vi "만도 소켓.vi"() -> ()   [LabVIEW 2023]
panel:
  out "array w/ subset deleted":dbl[](array[numeric])
  in  "Boolean":bool
  out "오차 각도":dbl
  out "x 교차점":dbl
  in  "stop":bool
  out "data out":string="99,99,0,0,0,0"
  out "전체 Array":dbl[](array[numeric])=[99.0, 99.0, 0.0, 0.0, 0.0, 0.0]
  out "빨간불":bool
  out "좌회전":bool
  out "직진":bool
  out "신호등 Array":dbl[](array[numeric])=[99.0, 99.0]
  out "생산자 FPS":dbl=111.11111111111111 format="%#_2g"
  out "error out":errorcluster
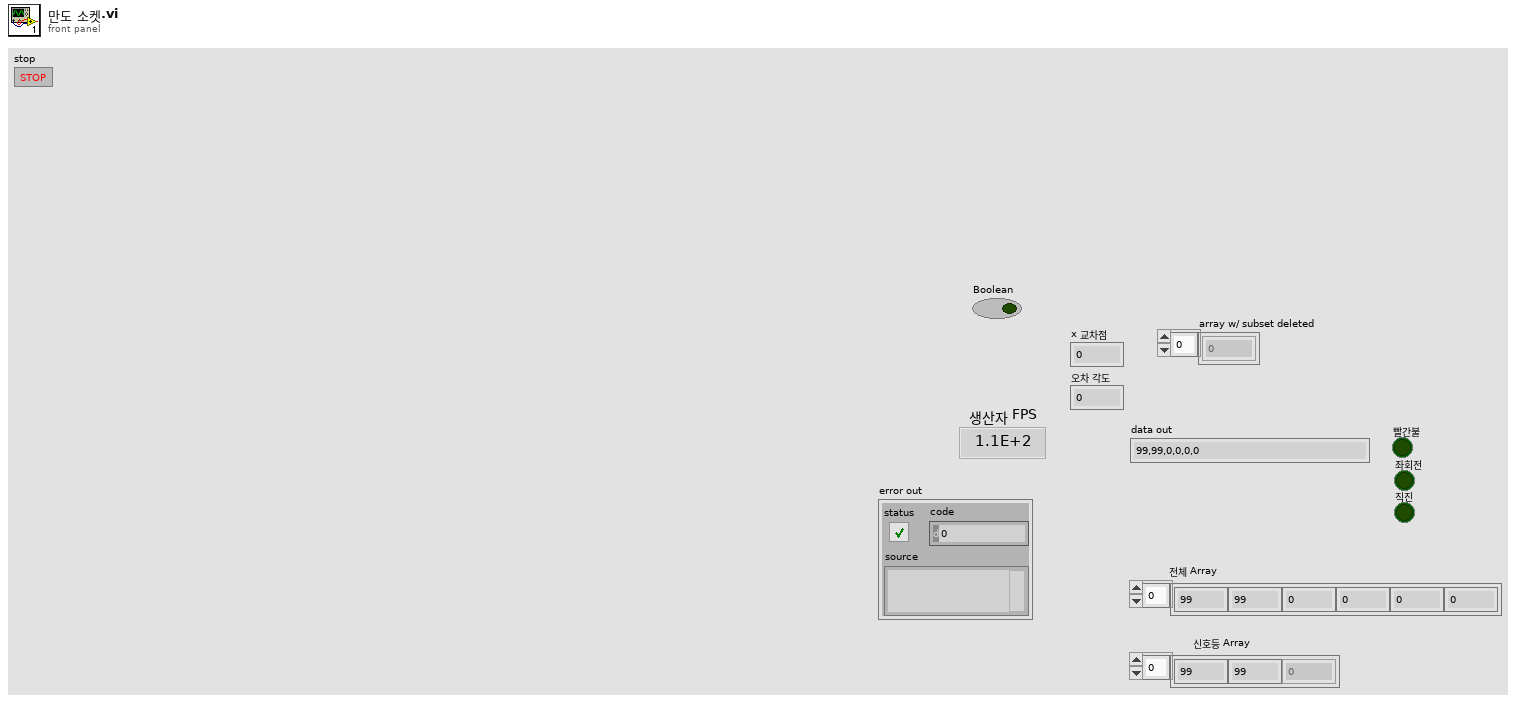
[diagram p1: front panel]
types:
  T1 = cluster{"빨간불":bool, "좌회전":bool, "직진":bool, "x 교차점":dbl, "오차 각도":dbl}
  T2 = enum16{"Standard", "Buffered", "CRLF", "Immediate"}
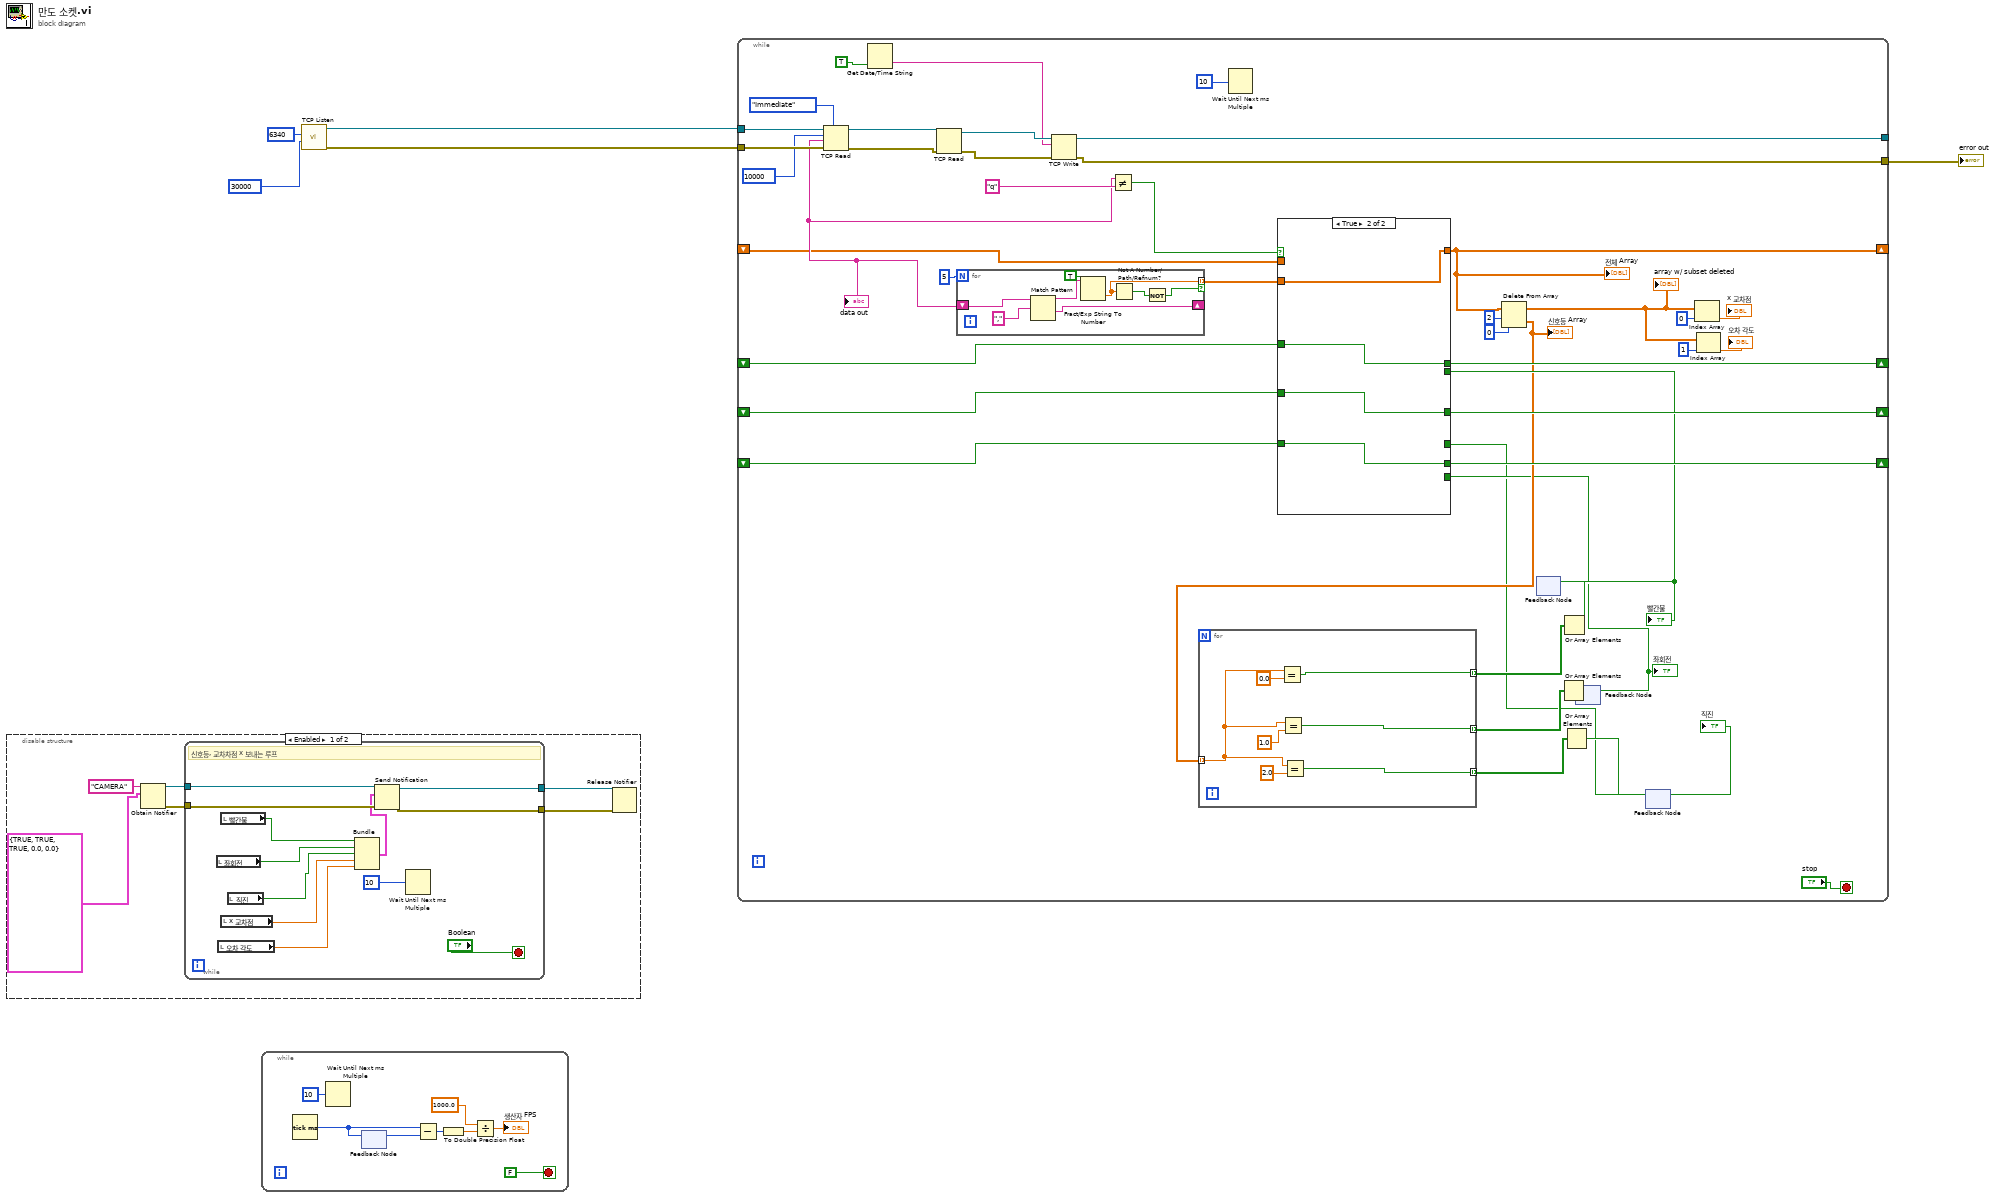
[diagram p0: block diagram]
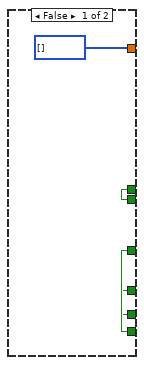
[diagram p2: hidden frame]
diagram:
  n1 = disable-structure shown="Enabled" {
    frame Enabled {
      n2 = Obtain Notifier(name (unnamed)="CAMERA", notification data type=cluster{bool, bool, bool, dbl, dbl} {TRUE, TRUE, TRUE, 0.0, 0.0}) -> (notifier out=w11:refnum<notifier>, error out=w9:errorcluster)  [unwired: 2 in, 1 out]
      n3 = while {
        tunnel: w11 -> [w23]
        tunnel: w9 -> [w22]
        tunnel: [w21] -> w8
        tunnel: [w20] -> w7
        stop <- "Boolean" stop-if-true
        # "신호등, 교차차점 x 보내는 루프"
        n4 = local read "좌회전"() -> (w16:bool)
        n5 = local read "오차 각도"() -> (w13:dbl)
        n6 = local read "빨간불"() -> (w17:bool)
        n7 = local read "x 교차점"() -> (w14:dbl)
        n8 = local read "직진"() -> (w15:bool)
        n9 = Bundle("빨간불"=w17, "좌회전"=w16, "직진"=w15, "x 교차점"=w14, "오차 각도"=w13) -> (w12:T1)  [unwired: 1 in]
        n10 = Send Notification(notification=w12, notifier=w23, error in (no error)=w22) -> (notifier out=w21:refnum<notifier>, error out=w20:errorcluster)
        n11 = Wait Until Next ms Multiple(millisecond multiple=u32 10 ("milliseconds to wait")) -> ()  [unwired: 1 out]
      }
      n12 = Release Notifier(notifier=w8, error in (no error)=w7) -> ()  [unwired: 1 in, 3 out]
    }
    frame Disabled {
    }
  }
  n13 = while {
    stop <- FALSE stop-if-true
    n14 = Tick Count (ms)() -> (millisecond timer value=w29:u32)
    n15 = Wait Until Next ms Multiple(millisecond multiple=u32 10 ("ms 배수")) -> ()  [unwired: 1 out]
    n16 = feedback #1() -> (w30:u32)  [unwired: 1 in]
    n17 = feedback-in #1(w29) -> ()
    n18 = Subtract(x=w29, y=w30) -> (x-y=w31:u32)
    n19 = To Double Precision Float(number=w31) -> (double precision float=w28:dbl)
    n20 = Divide(x=1000.0, y=w28) -> (x/y=→"생산자 FPS":dbl)
  }
  n21 = call <vilib>:"TCP Listen.vi"("timeout ms (wait forever: -1)"=30000, "port"=u16 6340) -> ("error out"=w2:errorcluster, "connection ID"=w3:refnum<k5>)  [unwired: 5 in, 3 out]
  n22 = while {
    tunnel: w3 -> [w75]
    tunnel: w2 -> [w74]
    tunnel: [w65] -> w1
    tunnel: [w64] -> _
    shift-right: [w42] -> _
    shift-left: _ -> [w50]
    shift-right: [w61] -> _
    shift-left: _ -> [w60]
    shift-right: [w59] -> _
    shift-left: _ -> [w58]
    shift-right: [w57] -> _
    shift-left: _ -> [w56]
    stop <- "stop" stop-if-true
    n23 = TCP Read(connection ID=w75, bytes to read=10000, error in (no error)=w74, 7:T2."Immediate" ("mode (standard)")) -> (connection ID out=w71:refnum<k5>, data out=w51:string, error out=w70:errorcluster)  [unwired: 1 in]
    "data out" <- w51
    n24 = Get Date/Time String(want seconds? (F)=TRUE) -> (time string=w66:string)  [unwired: 2 in, 1 out]
    n25 = TCP Read(connection ID=w71, error in (no error)=w70) -> (connection ID out=w69:refnum<k5>, error out=w68:errorcluster)  [unwired: 3 in, 1 out]
    n26 = for {
      N: 5 -> [_]
      tunnel: [w84] -> w53 mode=indexing if=w86
      shift-right: [w88] -> _
      shift-left: w51 -> [w90]
      n27 = Match Pattern(string=w90, regular expression=",") -> (before substring=w85:string, after substring=w88:string)  [unwired: 1 in, 2 out]
      n28 = Fract/Exp String To Number(use system decimal point (T)=TRUE, string=w85) -> (number=w84:dbl)  [unwired: 2 in, 1 out]
      n29 = Not A Number/Path/Refnum?(number/path/refnum=w84) -> (NaN/Path/Refnum?=w87:bool)
      n30 = Not(x=w87) -> (.not. x?=w86:bool)
    }
    n31 = TCP Write(connection ID=w69, data in=w66, error in (no error)=w68) -> (connection ID out=w64:refnum<k5>, error out=w65:errorcluster)  [unwired: 1 in, 1 out]
    n32 = Not Equal?(x=w51, y="q") -> (x != y?=w54:bool)
    n33 = Wait Until Next ms Multiple(millisecond multiple=u32 10) -> ()  [unwired: 1 out]
    n34 = feedback #2() -> (w45:bool)  [unwired: 1 in]
    "빨간불" <- w45
    n35 = feedback #3() -> (w38:bool)  [unwired: 1 in]
    "좌회전" <- w38
    n36 = feedback #4() -> (w32:bool)  [unwired: 1 in]
    "직진" <- w32
    n37 = case shown="True" w54 {
      tunnel: w53 -> [_ w95]
      tunnel: [w93 w98] -> w61
      tunnel: w60 -> [_ w98]
      tunnel: [w92 w97] -> w59
      tunnel: w58 -> [_ w97]
      tunnel: [w91 w96] -> w57
      tunnel: w56 -> [_ w96]
      tunnel: w50 -> [_ _]
      tunnel: [i32[] [] w95] -> w42
      tunnel: w45 -> [w93 _]
      tunnel: w38 -> [w92 _]
      tunnel: w32 -> [w91 _]
      frame False {
      }
      frame True {
      }
    }
    "전체 Array" <- w42
    n38 = Delete From Array(array=w42, length=2, index=0) -> (deleted portion=w39:dbl[], array with subset deleted=w37:dbl[])
    "신호등 Array" <- w39
    "array w/ subset deleted" <- w37
    n39 = for {
      tunnel: w39 -> [w80] mode=indexing
      tunnel: [w78] -> w49 mode=indexing
      tunnel: [w77] -> w48 mode=indexing
      tunnel: [w76] -> w47 mode=indexing
      n40 = Equal?(x=w80, y=0.0) -> (x = y?=w78:bool)
      n41 = Equal?(x=w80, y=1.0) -> (x = y?=w77:bool)
      n42 = Equal?(x=w80, y=2.0) -> (x = y?=w76:bool)
    }
    n43 = Or Array Elements(Boolean array=w48) -> (logical OR=w44:bool)
    n44 = Or Array Elements(Boolean array=w49) -> (logical OR=w46:bool)
    n45 = feedback-in #2(w46) -> ()
    n46 = Or Array Elements(Boolean array=w47) -> (logical OR=w43:bool)
    n47 = feedback-in #3(w44) -> ()
    n48 = feedback-in #4(w43) -> ()
    n49 = Index Array(array=w37, index=0) -> (element=→"x 교차점":dbl)
    n50 = Index Array(array=w37, index=1) -> (element=→"오차 각도":dbl)
  }
  "error out" <- w1
